vi "Test 5 Evaluate Card with Multiple Whitespace in Header.vi"(8 "error in (no error)":errorcluster, 11 "Test Case In":refnum<class "Card evaluator Test.lvclass">) -> (0 "error out":errorcluster, 3 "Test Case Out":refnum<class "Card evaluator Test.lvclass">)   [LabVIEW 2020, in "Card evaluator Test.lvclass"]
uses:
  Card evaluator Test.lvclass
  C:/Program Files (x86)/National Instruments/LabVIEW 2020/vi.lib/Astemes/LUnit/Test Case.lvclass
  <vilib>/Astemes/LUnit/Test Case.lvclass/Test Case.ctl
  4993e8ee-a06a-463a-9684-69129f64d5ce.vi
  <vilib>/Astemes/LUnit/Append Pass Result.vi
  <vilib>/Astemes/LUnit/Append Fail Result.vi
  <vilib>/Astemes/LUnit/Describe Comparison.vi
  <vilib>/Astemes/LUnit/Compare Variants.vi
  <vilib>/Astemes/LUnit/Variant to string.vi
  <vilib>/Utility/Data Type/Get Type Information.vi
  <vilib>/Utility/LVClass/Get LV Class Name.vi
  Card/Card.lvclass
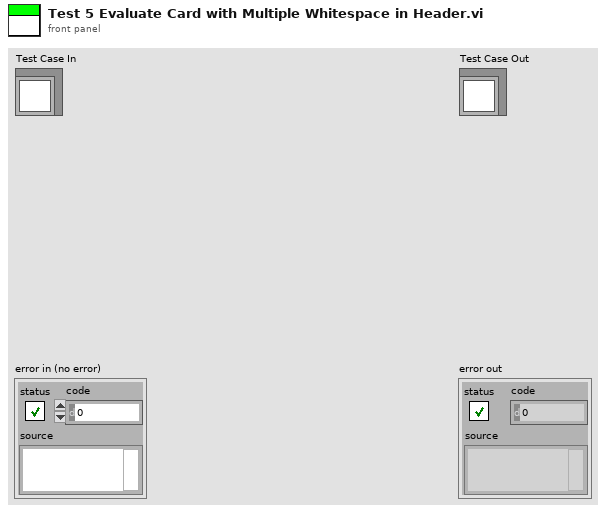
[diagram p1: front panel]
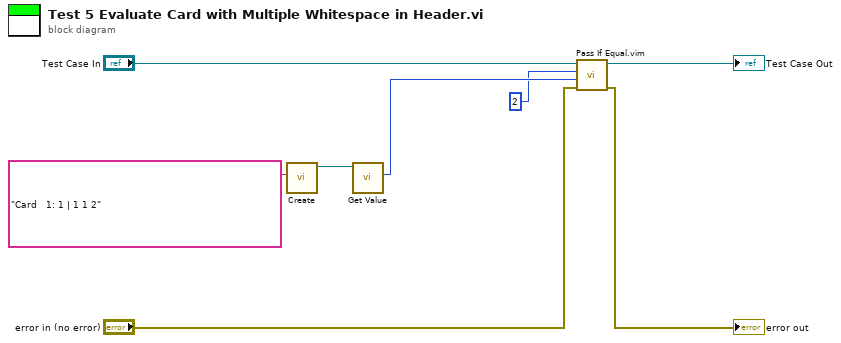
[diagram p0: block diagram]
diagram:
  n1 = call "Create.vi"("Card"="Card   1: 1 | 1 1 2") -> ("Card"=w3:refnum<class "Card.lvclass">)  [unwired: 9 in, 1 out]
  n2 = call-dynamic "Get Value.vi"("Card in"=w3) -> ("Value"=w2:i32)  [unwired: 8 in, 2 out]
  n3 = call "Pass If Equal.vim"("error in (no error)"="error in (no error)", "Actual"=w2, "Expected"=2 ("Value"), "LUnit Test Case In"="Test Case In") -> ("error out"=→"error out":errorcluster, "LUnit Test Case Out"=→"Test Case Out":refnum<class "Card evaluator Test.lvclass">)  [unwired: 6 in]
